vi "TDMS SN MN Escape Characters.vi"(1 "string":string) -> (0 "url-encoded string":string)   [LabVIEW 2011]
doc: "Encodes characters in URL format, replacing all characters except for alphanumeric and underscore with %xx, where xx is the hexadecimal value of the character."
panel:
  out "unsigned byte array":u8[](array[numeric])
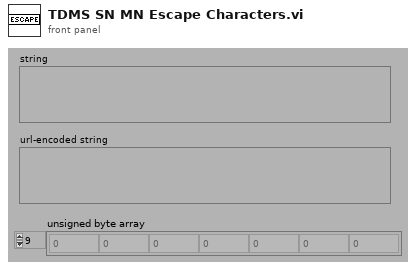
[diagram p1: front panel]
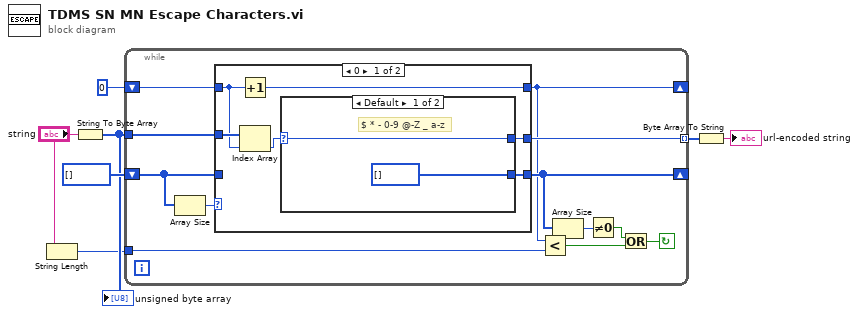
[diagram p0: block diagram]
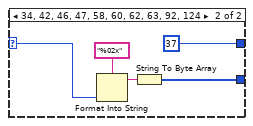
[diagram p2: hidden frame]
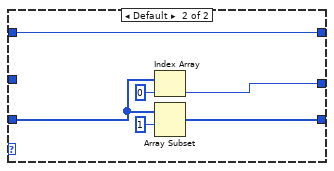
[diagram p3: hidden frame]
diagram:
  n1 = String Length(string="string") -> (length=w3:i32)
  n2 = String To Byte Array(string="string") -> (unsigned byte array=w5:u8[])
  "unsigned byte array" <- w5
  n3 = while {
    tunnel: w3 -> [w15]
    shift-left: 0 ("offset past match") -> [w9]
    shift-right: [w8] -> _
    tunnel: [w17] -> w4 mode=indexing
    tunnel: w5 -> [w16]
    shift-left: u8[] [] ("Array Constant") -> [w18]
    shift-right: [w11] -> _
    stop <- w10 continue-if-true
    n4 = Array Size(array=w18) -> (size(s)=w19:i32)
    n5 = case shown="0" w19 {
      tunnel: w18 -> [_ w38]
      tunnel: [w21 w33] -> w11
      tunnel: [w23 w35] -> w17
      tunnel: w16 -> [w25 _]
      tunnel: w9 -> [w20 w34]
      tunnel: [w22 w34] -> w8
      frame 0 {
        n6 = Increment(x=w20) -> (x+1=w22:i32)
        n7 = Index Array(array=w25, index=w20) -> (element=w24:u8)
        n8 = case shown="Default" w24 {
          selector: w24 -> [w27 w31]
          tunnel: [w27 u8 37] -> w23
          tunnel: [u8[] [] ("Array Constant") w29] -> w21
          frame Default {
            # "$ * - 0-9 @-Z _ a-z"
          }
          frame 34, 42, 46, 47, 58, 60, 62, 63, 92, 124 {
            n9 = Format Into String(format string="%02x", w31) -> (resulting string=w28:string)  [unwired: 2 in, 1 out]
            n10 = String To Byte Array(string=w28) -> (unsigned byte array=w29:u8[])
          }
        }
      }
      frame Default {
        n11 = Index Array(array=w38, index=0 ("Index")) -> (element=w35:u8)
        n12 = Array Subset(array=w38, index=1 ("Array Index")) -> (w33:u8[])  [unwired: 1 in]
      }
    }
    n13 = Less?(x=w8, y=w15) -> (x < y?=w12:bool)
    n14 = Array Size(array=w11) -> (size(s)=w13:i32)
    n15 = Not Equal To 0?(x=w13) -> (x != 0?=w14:bool)
    n16 = Or(x=w14, y=w12) -> (x .or. y?=w10:bool)
  }
  n17 = Byte Array To String(unsigned byte array=w4) -> (string=→"url-encoded string":string)
